vi "MH_CalcDeltaTB.vi"(0 "Buffindex":i32, 1 "TrueTime":u64, 3 "Buffsize":i32, 5 "Data In":u64[](array[numeric]), 7 "DeltasBuffer":i32[](array[numeric]), 9 "Deltaindex":i32, 11 "DBuffSize":i32=10, 12 "WinIndex":i32, 13 "WIndowW":i32) -> (4 "Write Delta":bool, 6 "NewDelta":bool, 8 "DeltasBufferOut":i32[](array[numeric]), 10 "DeltaIndexOut":i32, 14 "WinIndexOut":i32, 15 "DBuffSize out":i32=10)   [LabVIEW 2019]
panel:
  # "here"
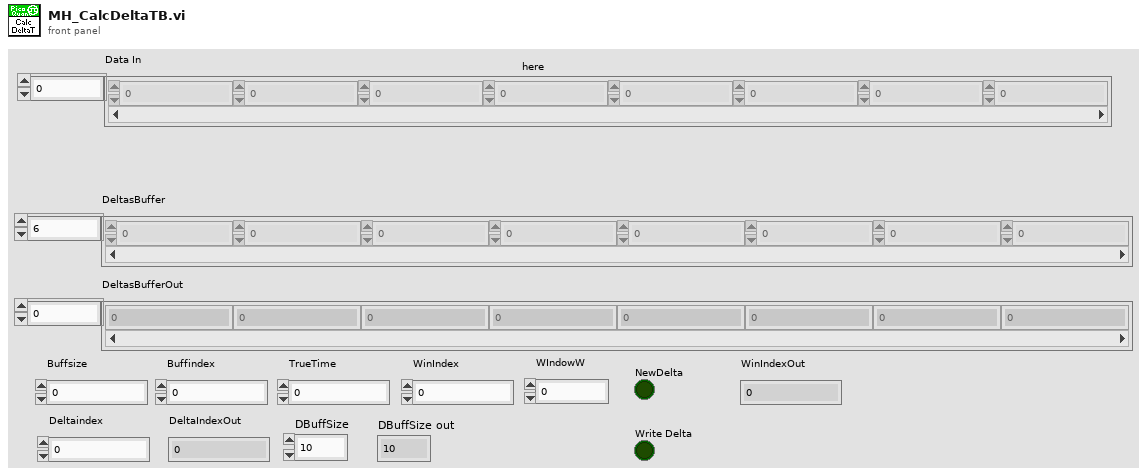
[diagram p1: front panel]
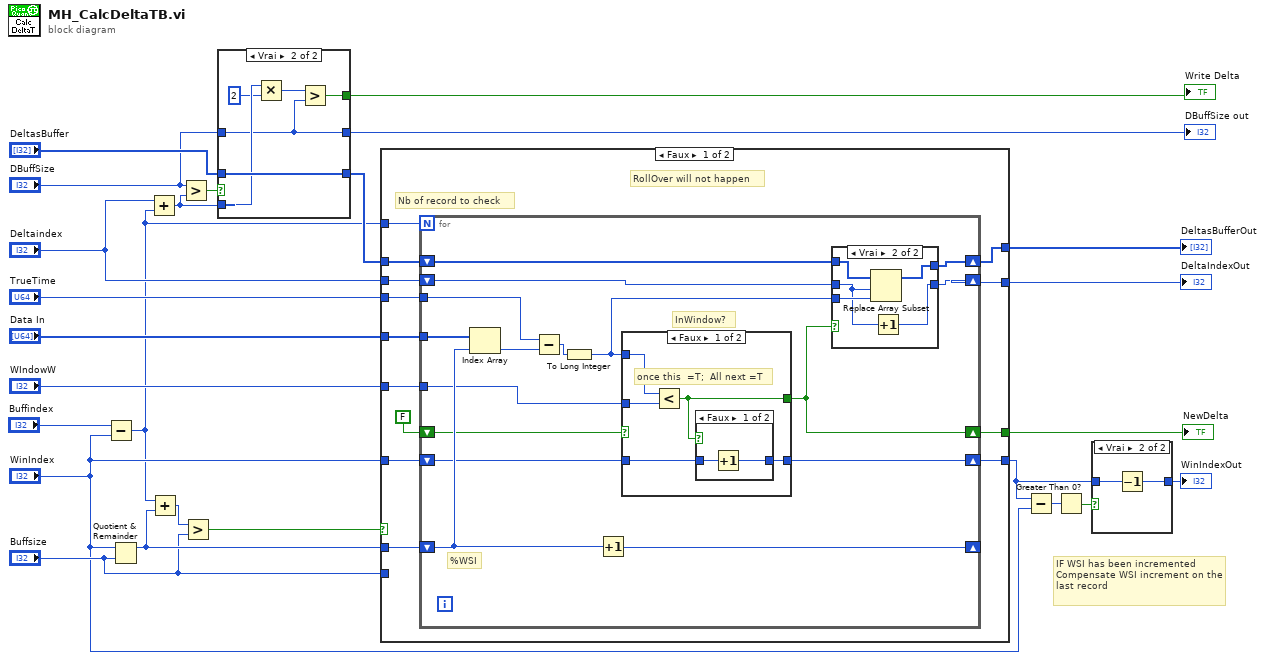
[diagram p0: block diagram]
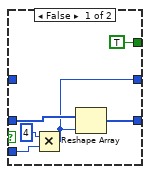
[diagram p2: hidden frame]
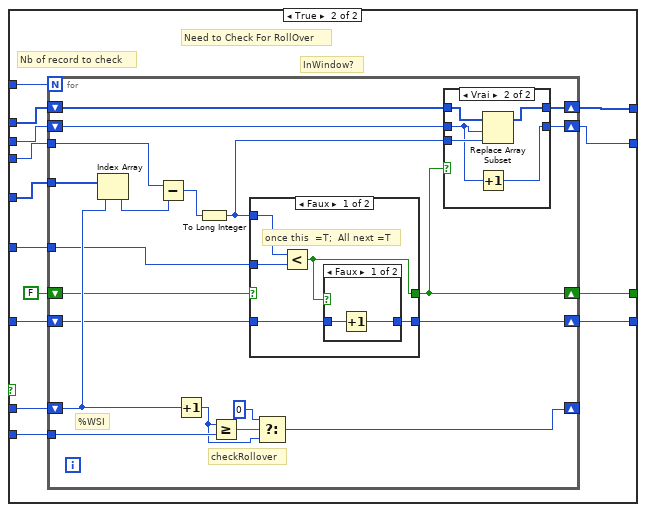
[diagram p6: hidden frame]
diagram:
  # "IF WSI has been incremented\nCompensate WSI increment on the last record"
  n1 = Subtract(x="Buffindex", y="WinIndex") -> (x-y=w1:i32)
  n2 = Quotient & Remainder(x="WinIndex", y="Buffsize") -> (x-y*floor(x/y)=w17:i32)  [unwired: 1 out]
  n3 = Add(x="Deltaindex", y=w1) -> (x+y=w7:i32)
  n4 = Add(x=w1, y=w17) -> (x+y=w16:i32)
  n5 = Greater?(x="DBuffSize", y=w7) -> (0:w10:bool)
  n6 = Greater?(x=w16, y="Buffsize") -> (0:w14:bool)
  n7 = case shown="Vrai" w10 {
    tunnel: [w30 w37] -> w8
    tunnel: "DeltasBuffer" -> [w31 w37]
    tunnel: w7 -> [w29 w36]
    tunnel: [w27 w33] -> w6
    tunnel: "DBuffSize" -> [_ w33]
    tunnel: [TRUE w32] -> w3
    frame False {
      n8 = Multiply(x=4, y=w29) -> (x*y=w27:i32)
      n9 = Reshape Array(w31, w27) -> (w30:i32[])
    }
    frame True {
      n10 = Multiply(x=w36, y=2) -> (x*y=w35:i32)
      n11 = Greater?(x=w35, y=w33) -> (0:w32:bool)
    }
  }
  "DBuffSize out" <- w6
  "Write Delta" <- w3
  n12 = case shown="Faux" w14 {
    tunnel: "Data In" -> [w50 w97]
    tunnel: "TrueTime" -> [w49 w96]
    tunnel: "WIndowW" -> [w48 w95]
    tunnel: [w47 w94] -> w22
    tunnel: "WinIndex" -> [w45 w92]
    tunnel: [w44 w91] -> w18
    tunnel: w1 -> [w43 w90]
    tunnel: w17 -> [w42 w89]
    tunnel: "Buffsize" -> [_ w88]
    tunnel: w8 -> [w41 w87]
    tunnel: "Deltaindex" -> [w40 w86]
    tunnel: [w38 w85] -> w13
    tunnel: [w39 w84] -> w12
    frame False {
      # "RollOver will not happen"
      # "Nb of record to check"
      n13 = for {
        N: w43 -> [_]
        tunnel: w50 -> [w66]
        tunnel: w49 -> [w57]
        shift-right: [w60] -> w44
        shift-left: w45 -> [w61]
        shift-right: [w59] -> _
        shift-left: w42 -> [w64]
        tunnel: w48 -> [w63]
        shift-right: [w51] -> w47
        shift-left: FALSE -> [w62]
        shift-right: [w53] -> w38
        shift-left: w41 -> [w56]
        shift-right: [w52] -> w39
        shift-left: w40 -> [w55]
        # "InWindow?"
        # "%WSI"
        n14 = Index Array(array=w66, index=w64) -> (element=w58:u64)
        n15 = Subtract(x=w57, y=w58) -> (x-y=w65:u64)
        n16 = To Long Integer(number=w65) -> (32bit integer=w54:i32)
        n17 = Increment(x=w64) -> (x+1=w59:i32)
        n18 = case shown="Faux" w62 {
          selector: w62 -> [_ w82]
          tunnel: w54 -> [w78 _]
          tunnel: w63 -> [w77 _]
          tunnel: [w74 w82] -> w51
          tunnel: w61 -> [w76 w83]
          tunnel: [w75 w83] -> w60
          frame False {
            # "once this  =T;  All next =T"
            n19 = Less?(x=w78, y=w77) -> (x < y?=w74:bool)
            n20 = case shown="Faux" w74 {
              tunnel: w76 -> [w80 w81]
              tunnel: [w79 w81] -> w75
              frame False {
                n21 = Increment(x=w80) -> (x+1=w79:i32)
              }
              frame True {
              }
            }
          }
          frame True {
          }
        }
        n22 = case shown="Vrai" w51 {
          tunnel: w56 -> [w68 w70]
          tunnel: w54 -> [_ w73]
          tunnel: w55 -> [w67 w69]
          tunnel: [w67 w72] -> w52
          tunnel: [w68 w71] -> w53
          frame False {
          }
          frame True {
            n23 = Replace Array Subset(array=w70, new element=w73, index=w69) -> (w71:i32[])
            n24 = Increment(x=w69) -> (x+1=w72:i32)
          }
        }
      }
    }
    frame True {
      # "InWindow?"
      # "Need to Check For RollOver"
      # "Nb of record to check"
      n25 = for {
        N: w90 -> [_]
        tunnel: w97 -> [w117]
        tunnel: w96 -> [w104]
        shift-right: [w110] -> w91
        shift-left: w92 -> [w111]
        shift-right: [w114] -> _
        shift-left: w89 -> [w115]
        tunnel: w88 -> [w116]
        tunnel: w95 -> [w113]
        shift-right: [w100] -> w94
        shift-left: FALSE -> [w112]
        shift-right: [w103] -> w85
        shift-left: w87 -> [w101]
        shift-right: [w102] -> w84
        shift-left: w86 -> [w99]
        # "checkRollover"
        # "%WSI"
        n26 = Index Array(array=w117, index=w115) -> (element=w105:u64)
        n27 = Subtract(x=w104, y=w105) -> (x-y=w106:u64)
        n28 = Increment(x=w115) -> (x+1=w107:i32)
        n29 = To Long Integer(number=w106) -> (32bit integer=w98:i32)
        n30 = Greater Or Equal?(x=w107, y=w116) -> (x >= y?=w109:bool)
        n31 = case shown="Faux" w112 {
          selector: w112 -> [_ w133]
          tunnel: w98 -> [w129 _]
          tunnel: w113 -> [w128 _]
          tunnel: [w125 w133] -> w100
          tunnel: w111 -> [w127 w134]
          tunnel: [w126 w134] -> w110
          frame False {
            # "once this  =T;  All next =T"
            n32 = Less?(x=w129, y=w128) -> (x < y?=w125:bool)
            n33 = case shown="Faux" w125 {
              tunnel: w127 -> [w131 w132]
              tunnel: [w130 w132] -> w126
              frame False {
                n34 = Increment(x=w131) -> (x+1=w130:i32)
              }
              frame True {
              }
            }
          }
          frame True {
          }
        }
        n35 = Select(t=0 ("x+1"), s=w109, f=w107) -> (s? t:f=w114:i32)
        n36 = case shown="Vrai" w100 {
          tunnel: w101 -> [w119 w121]
          tunnel: w98 -> [_ w124]
          tunnel: w99 -> [w118 w120]
          tunnel: [w118 w123] -> w102
          tunnel: [w119 w122] -> w103
          frame False {
          }
          frame True {
            n37 = Increment(x=w120) -> (x+1=w123:i32)
            n38 = Replace Array Subset(array=w121, new element=w124, index=w120) -> (w122:i32[])
          }
        }
      }
    }
  }
  "NewDelta" <- w22
  "DeltasBufferOut" <- w13
  "DeltaIndexOut" <- w12
  n39 = Subtract(x=w18, y="WinIndex") -> (x-y=w21:i32)
  n40 = Greater Than 0?(x=w21) -> (x > 0?=w20:bool)
  n41 = case shown="Vrai" w20 {
    tunnel: [w135 w136] -> w19
    tunnel: w18 -> [w135 w137]
    frame False {
    }
    frame True {
      n42 = Decrement(x=w137) -> (x-1=w136:i32)
    }
  }
  "WinIndexOut" <- w19
